vi "TTA_MATLAB_Tile_Set_PA_Control_Corr_Status.vi"(0 "Channels":string[](array[combo]), 5 "ModeAdapt":string(combo), 11 "error in":errorcluster) -> (4 "Success":bool, 6 "TileSuccessComm":bool[](array[boolean]), 8 "TileSuccessOp":bool[](array[boolean]), 15 "error out":errorcluster)   [LabVIEW 2016]
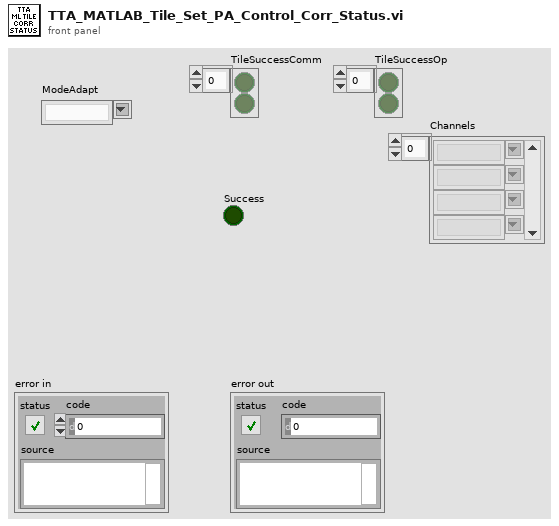
[diagram p1: front panel]
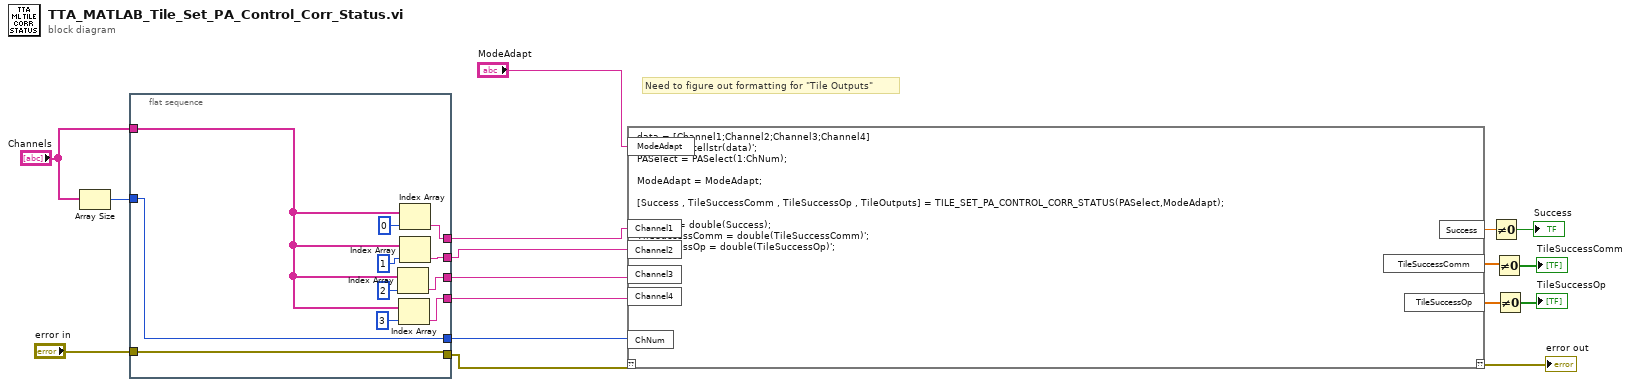
[diagram p0: block diagram]
diagram:
  # "Need to figure out formatting for \"Tile Outputs\""
  n1 = Array Size(array="Channels") -> (size(s)=w9:i32)
  n2 = flat-sequence {
    tunnel: "error in" -> [w28]
    tunnel: [w27] -> w5
    tunnel: w9 -> [w21]
    tunnel: [w28] -> w7
    tunnel: "Channels" -> [w20]
    tunnel: [w24] -> w4
    tunnel: [w22] -> w3
    tunnel: [w21] -> w6
    tunnel: [w18] -> w2
    frame #0 {
      n3 = Index Array(array=w20, index=2) -> (element=w22:string)
      n4 = Index Array(array=w20, index=3) -> (element=w18:string)
      n5 = Index Array(array=w20, index=0) -> (element=w27:string)
      n6 = Index Array(array=w20, index=1) -> (element=w24:string)
    }
  }
  n7 = script code="data = [Channel1;Channel2;Channel3;Channel4]\nPASelect = cellstr(data)';\nPASelect = PASelect(1:ChNum);\n\nModeAdapt = ModeAdapt;\n\n[Success , TileSuccessComm , TileSuccessOp , TileOutputs] = TILE_SET_PA_CONTROL_CORR_STATUS(PASelect,ModeAdapt);\n\nSuccess = double(Success);\nTileSuccessComm = double(TileSuccessComm)';\nTileSuccessOp = double(TileSuccessOp)';"("??"=w7, "Channel1"=w5, "ModeAdapt"="ModeAdapt", "ChNum"=w6, "Channel2"=w4, "Channel3"=w3, "Channel4"=w2) -> ("??"=→"error out":errorcluster, "Success"=w16:dbl, "TileSuccessComm"=w14:dbl[], "TileSuccessOp"=w12:dbl[])
  n8 = Not Equal To 0?(x=w16) -> (x != 0?=→"Success":bool)
  n9 = Not Equal To 0?(x=w14) -> (x != 0?=→"TileSuccessComm":bool[])
  n10 = Not Equal To 0?(x=w12) -> (x != 0?=→"TileSuccessOp":bool[])
